vi "Power Accuracy Configuration.vi"(6 "Write? (f)":bool, 7 "Connection Refnum":T2, 8 "error in (no error)":errorcluster, 9 "Configuration (\"\")":string, 11 "Template Keys (empty)":T1) -> (0 "error out":errorcluster, 1 "Configuration":string, 3 "Template Keys":T1, 5 "Connection Refnum":T2)   [LabVIEW 2011]
uses:
  Summitek EXT/ODBC/SQL Controls/Connection Refnum.ctl
  ITK EXT/utils/keyedarr.llb/Keyed Array.ctl
  ITK EXT/utils/strutil.llb/Case Matching.ctl
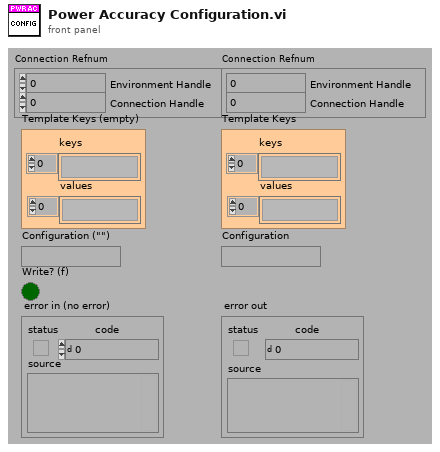
[diagram p1: front panel]
types:
  T1 = typedef "Keyed Array.ctl" = cluster{"keys":string[], "values":string[]}
  T2 = typedef "Connection Refnum.ctl" = cluster{"Environment Handle":i32, "Connection Handle":i32}
  T3 = typedef "Case Matching.ctl" = enum16{"a != A", "a == A", "system"}
  T4 = typedef "Power Accuracy Test Parameters.ctl" = cluster{"Stimulus":T5, "Measurement":T6, "Display":T9, "Limit":T10, "Calibration":T11}
  T5 = typedef "Power Accuracy Stimulus Parameters.ctl" = cluster{"Power Start":i32, "Power Stop":i32, "Frequency Type":enum16{"Band Edges", "Custom"}, "Frequency Points":dbl[], "TX 1 Frequency (MHz)":cluster{"Min":dbl, "Max":dbl}, "TX 2 Frequency (MHz)":cluster{"Min":dbl, "Max":dbl}, "RX Frequency (MHz)":cluster{"Min":dbl, "Max":dbl}, "Pad Model Number":string, "Pad Serial Number":string, "Pad Values":dbl[][][]}
  T6 = typedef "Power Accuracy Measurement Parameters.ctl" = cluster{"DUT Port":T7, "Direction":T8}
  T7 = typedef "DUTport.ctl" = enum16{"Port 1", "Port 2"}
  T8 = typedef "MeasMode.ctl" = u16
  T9 = typedef "Power Accuracy Display Parameters.ctl" = cluster{"Power":cluster{"Min":i32, "Max":i32}, "Tolerance":cluster{"Min":dbl, "Max":dbl}}
  T10 = typedef "Power Accuracy Limit Parameters.ctl" = cluster{"Tolerance":dbl}
  T11 = typedef "Power Accuracy Calibration State.ctl" = cluster{"Calibrated?":bool}
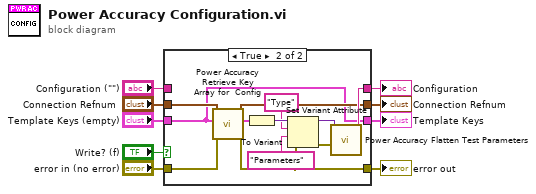
[diagram p0: block diagram]
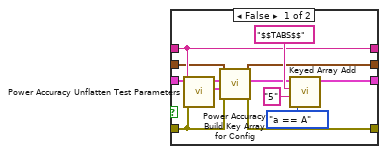
[diagram p2: hidden frame]
diagram:
  n1 = case shown="True" "Write? (f)" {
    tunnel: "error in (no error)" -> [w11 w27]
    tunnel: [w14 w22] -> w3
    tunnel: "Template Keys (empty)" -> [w12 w22]
    tunnel: "Configuration (\"\")" -> [w18 _]
    tunnel: [w13 w26] -> w2
    tunnel: [w18 w28] -> w5
    tunnel: "Connection Refnum" -> [w17 w25]
    tunnel: [w16 w24] -> w4
    frame False {
      n2 = call "Power Accuracy Unflatten Test Parameters.vi"("error in (no error)"=w11, "Parameter String"=w18) -> ("Power Accuracy Test Parameters"=w10:T4)  [unwired: 7 in, 2 out]
      n3 = call "Power Accuracy Build Key Array for Config.vi"("error in (no error)"=w11, "Power Accuracy Test Parameters"=w10, "Key Array In"=w12, "Connection Refnum"=w17) -> ("error out"=w13:errorcluster, "Key Array Out"=w15:T1, "Connection Refnum"=w16:T2)  [unwired: 5 in]
      n4 = call "Keyed Array Add.vi"("case matching (sensitive)"=Case_Matching."a == A", "value"="5", "key"="$$TABS$$", "array in"=w15) -> ("array out"=w14:T1)  [unwired: 3 out]
    }
    frame True {
      n5 = call "Power Accuracy Retrieve Key Array for  Config.vi"("error in (no error)"=w27, "Key Array In"=w22, "Connection Refnum"=w25) -> ("error out"=w26:errorcluster, "Power Accuracy Test Parameters"=w23:T4, "Connection Refnum"=w24:T2)  [unwired: 6 in]
      n6 = To Variant(anything=w23) -> (Variant=w33:variant)
      n7 = Set Variant Attribute(Variant=w33, name="Type", value="Parameters" ("name"), error in=w26) -> (Variant out=w29:variant, error out=w32:errorcluster)  [unwired: 1 out]
      n8 = call "Power Accuracy Flatten Test Parameters.vi"("error in (no error)"=w32, "Parameter Variant"=w29) -> ("Parameter String"=w28:string)  [unwired: 8 in, 1 out]
    }
  }
  "error out" <- w2
  "Connection Refnum" <- w4
  "Template Keys" <- w3
  "Configuration" <- w5
